vi "Client Connection Loop.vi"(11 "TCPMessaging in":refnum<class "TCPMessaging.lvclass">) -> ()   [LabVIEW 2020, in "Vecto.lvlib" / "TCPMessaging.lvclass"]
uses:
  TCPMessaging.lvclass
  Client Connection State.ctl
  TCPMessaging.lvclass/TCPMessaging.ctl
  EventLoggingService/EventLoggingService.lvclass/EventLoggingService.ctl
  Connection State.ctl
  <vilib>/Utility/error.llb/Error Cluster From Error Code.vi
  EventLogHandler/EventLogHandler.lvclass
  proto/TcpClientHello/TcpClientHello.lvlib
  Vecto.lvlib
  EventLoggingService/EventLoggingService.lvclass
  Connected Status.ctl
panel:
  out "State":T1
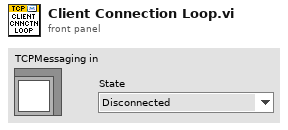
[diagram p1: front panel]
types:
  T1 = typedef "Vecto.lvlib/TCPMessaging.lvclass/Client Connection State.ctl" = enum16{"Disconnected", "Accept", "Notify Connect", "Wait Running", "Connected", "Notify Disconnect", "Reset", "Wait Stopped"}
  T2 = typedef "Vecto.lvlib/Connection State.ctl" = enum16{"Connected", "Disconnected"}
  T3 = typedef "Vecto.lvlib/Connected Status.ctl" = enum16{"Disconnected", "Connected", "Bad Config", "Not Allowed", "Server"}
  T4 = typedef "TcpClientHello.lvlib/Data.ctl" = cluster{"node_id":u32, "system":string, "cluster":string, "node_name":string, "app_version":string, "config_version":string, "config_hash":string, "node_alias":string}
  T5 = typedef "ConnectStatus.lvlib/Enumeration.ctl" = enum16{"STATUS_UNKNOWN", "STATUS_SUCCESS", "STATUS_ERROR", "STATUS_BAD_CONFIG", "STATUS_BAD_SYSTEM", "STATUS_BAD_CLUSTER", "STATUS_NOT_ALLOWED"}
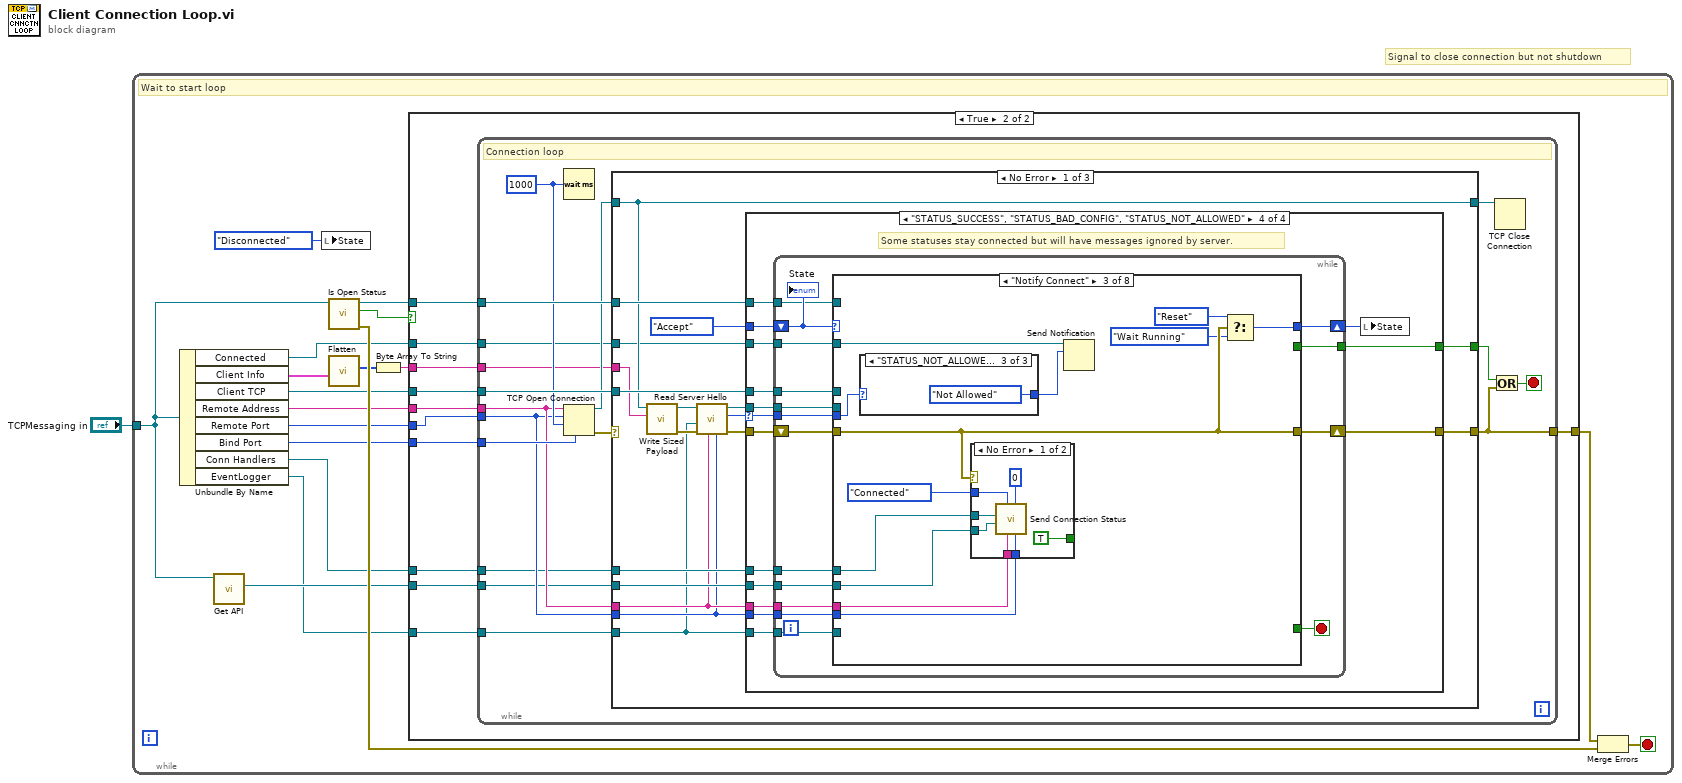
[diagram p0: block diagram]
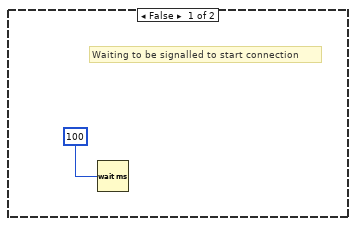
[diagram p2: hidden frame]
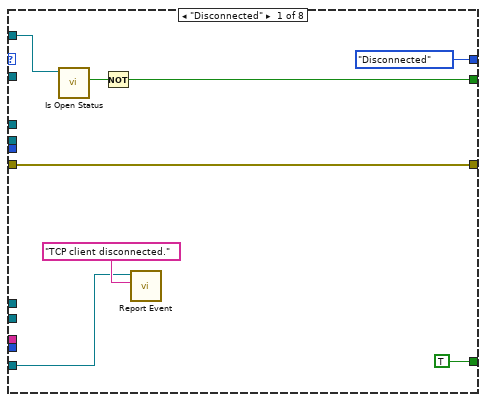
[diagram p6: hidden frame]
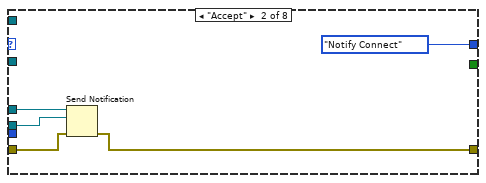
[diagram p7: hidden frame]
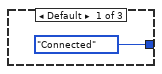
[diagram p8: hidden frame]
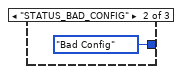
[diagram p9: hidden frame]
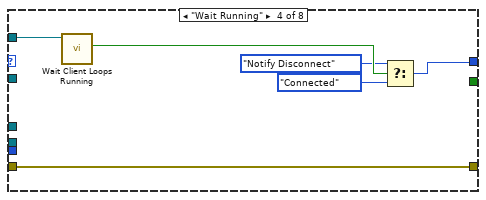
[diagram p11: hidden frame]
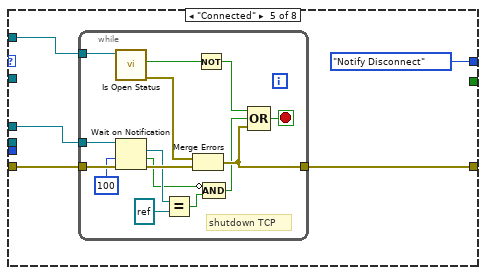
[diagram p12: hidden frame]
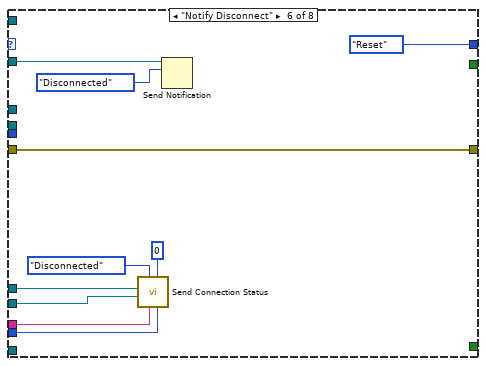
[diagram p13: hidden frame]
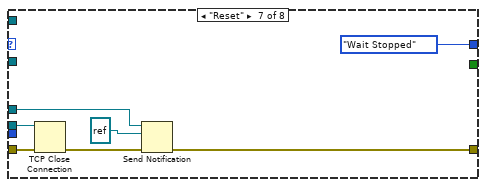
[diagram p14: hidden frame]
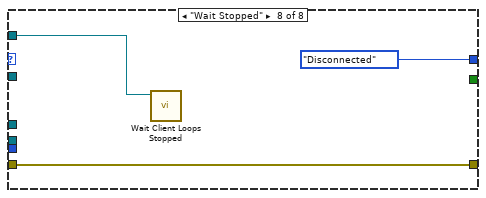
[diagram p15: hidden frame]
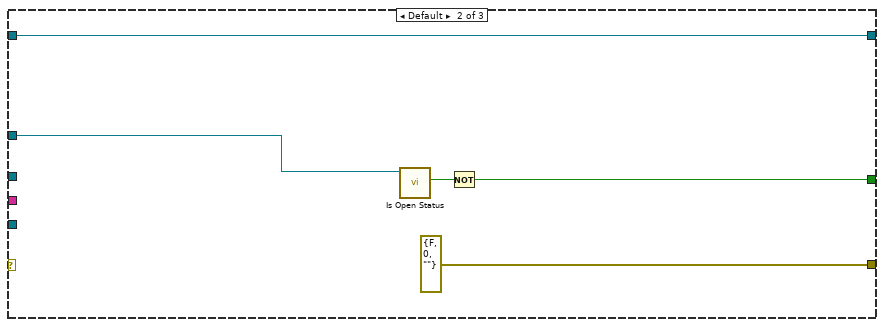
[diagram p16: hidden frame]
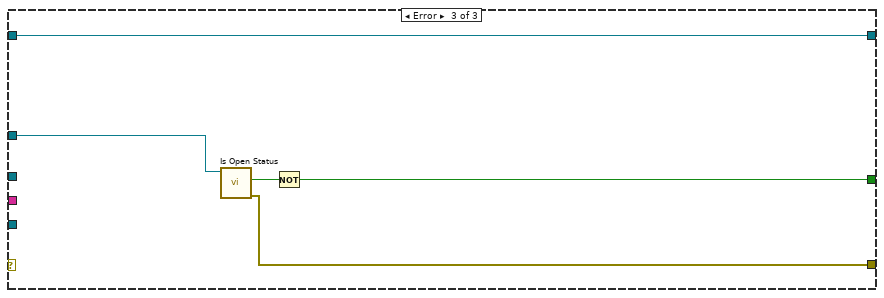
[diagram p17: hidden frame]
diagram:
  # "Signal to close connection but not shutdown"
  n1 = while {
    tunnel: "TCPMessaging in" -> [w6]
    stop <- w8 stop-if-true
    # "Wait to start loop"
    n2 = Unbundle By Name(w6) -> ("Connected"=w2:refnum<notifier>, "Client Info"=w5:T4, "Client TCP"=w13:refnum<notifier>, "Remote Address"=w18:string, "Remote Port"=w17:u16, "Bind Port"=w14:u16, "Conn Handlers"=w10:refnum<queue>, "EventLogger"=w4:refnum<class "EventLoggingService.lvclass">)
    n3 = call "Get API.vi"("TCPMessaging in"=w6) -> ("TCP Messaging API"=w9:refnum<class "TCPMessageAPI.lvclass">)  [unwired: 8 in, 2 out]
    n4 = local write "State"(Client_Connection_State."Disconnected" ("State")) -> ()
    n5 = call "Is Open Status.vi"("TCPMessaging in"=w6) -> ("error out"=w19:errorcluster, "Open"=w15:bool, "TCPMessaging out"=w16:refnum<class "TCPMessaging.lvclass">)  [unwired: 8 in]
    n6 = call "Flatten.vi"("Data"=w5) -> ("Buffer"=w12:u8[])  [unwired: 9 in, 1 out]
    n7 = Byte Array To String(unsigned byte array=w12) -> (string=w11:string)
    n8 = case shown="True" w15 {
      tunnel: w18 -> [_ w28]
      tunnel: w17 -> [_ w29]
      tunnel: w16 -> [_ w31]
      tunnel: w14 -> [_ w30]
      tunnel: w13 -> [_ w27]
      tunnel: w11 -> [_ w26]
      tunnel: w10 -> [_ w25]
      tunnel: w9 -> [_ w24]
      tunnel: [_ w23] -> w7
      tunnel: w4 -> [_ w22]
      tunnel: w2 -> [_ w21]
      frame False {
        # "Waiting to be signalled to start connection"
        n9 = Wait (ms)(milliseconds to wait=u32 100) -> ()  [unwired: 1 out]
      }
      frame True {
        n10 = while {
          tunnel: w31 -> [w44]
          tunnel: w30 -> [w47]
          tunnel: w29 -> [w37]
          tunnel: w28 -> [w38]
          tunnel: w27 -> [w45]
          tunnel: w26 -> [w39]
          tunnel: w25 -> [w36]
          tunnel: w24 -> [w35]
          tunnel: w22 -> [w34]
          tunnel: [w33] -> w23
          tunnel: w21 -> [w32]
          stop <- w48 stop-if-true
          w40 = 1000 ("timeout ms (60000)")
          # "Connection loop"
          n11 = Wait (ms)(milliseconds to wait=w40) -> ()  [unwired: 1 out]
          n12 = TCP Open Connection(address=w38, remote port or service name=w37, timeout ms (60000)=w40, local port=w47) -> (connection ID=w42:refnum<k5>, error out=w46:errorcluster)  [unwired: 1 in]
          n13 = case shown="No Error" w46 {
            tunnel: w42 -> [w62 w185 w188]
            tunnel: w45 -> [w65 _ _]
            tunnel: w44 -> [w66 w184 w191]
            tunnel: [w59 errorcluster {"status"=FALSE, "code"=0, "source"=""} ("error IO") w187] -> w33
            tunnel: [w64 w182 w189] -> w43
            tunnel: [w62 w185 w188] -> w41
            tunnel: w39 -> [w63 _ _]
            tunnel: w38 -> [w53 _ _]
            tunnel: w37 -> [w52 _ _]
            tunnel: w36 -> [w61 _ _]
            tunnel: w35 -> [w60 _ _]
            tunnel: w34 -> [w51 _ _]
            tunnel: w32 -> [w49 _ _]
            frame No Error {
              n14 = call "Write Sized Payload.vi"("Payload"=w63, "TCP in"=w62) -> ("error out"=w57:errorcluster, "TCP"=w58:refnum<k5>)  [unwired: 8 in]
              n15 = call "Read Server Hello.vi"("Port"=w52, "Address"=w53, "error in (no error)"=w57, "EventLogger"=w51, "TCP in"=w58) -> ("error out"=w56:errorcluster, "status"=w54:T5, "TCP"=w55:refnum<k5>)  [unwired: 4 in]
              n16 = case shown="\"STATUS_SUCCESS\", \"STATUS_BAD_CONFIG\", \"STATUS_NOT_ALLOWED\"" w54 {
                selector: w54 -> [_ _ _ w70]
                tunnel: w66 -> [_ _ _ w76]
                tunnel: w65 -> [_ _ _ w78]
                tunnel: [_ _ _ w73] -> w64
                tunnel: w61 -> [_ _ _ w80]
                tunnel: w60 -> [_ _ _ w81]
                tunnel: w53 -> [_ _ _ w82]
                tunnel: w52 -> [_ _ _ w83]
                tunnel: [w67 w68 w69 w74] -> w59
                tunnel: w56 -> [w67 w68 w69 w79]
                tunnel: w55 -> [_ _ _ w77]
                tunnel: w51 -> [_ _ _ w84]
                tunnel: Client_Connection_State."Accept" ("Client Connection State") -> [_ _ _ w75]
                tunnel: w49 -> [_ _ _ w71]
                frame "STATUS_BAD_SYSTEM", "STATUS_BAD_CLUSTER" {
                  # "Requires app update to resolve."
                }
                frame "STATUS_UNKNOWN" {
                }
                frame "STATUS_ERROR" {
                  # "Unknown error on server side, retry after loop delay."
                }
                frame "STATUS_SUCCESS", "STATUS_BAD_CONFIG", "STATUS_NOT_ALLOWED" {
                  # "Some statuses stay connected but will have messages ignored by server."
                  n17 = while {
                    tunnel: w84 -> [w88]
                    tunnel: w83 -> [w89]
                    tunnel: w82 -> [w90]
                    tunnel: w81 -> [w91]
                    tunnel: w80 -> [w92]
                    shift-right: [w93] -> w74
                    shift-left: w79 -> [w94]
                    tunnel: w78 -> [w96]
                    tunnel: w77 -> [w95]
                    tunnel: w76 -> [w97]
                    shift-right: [w99] -> w72
                    shift-left: w75 -> [w100]
                    tunnel: [w87] -> w73
                    tunnel: w71 -> [w86]
                    tunnel: w70 -> [w85]
                    stop <- w98 stop-if-true
                    n18 = case shown="\"Notify Connect\"" w100 {
                      tunnel: [Client_Connection_State."Disconnected" ("Client Connection State") Client_Connection_State."Notify Connect" ("Client Connection State") w118 w136 Client_Connection_State."Notify Disconnect" ("Client Connection State") Client_Connection_State."Reset" ("Client Connection State") Client_Connection_State."Wait Stopped" ("Client Connection State") Client_Connection_State."Disconnected" ("Client Connection State")] -> w99
                      tunnel: [TRUE _ _ _ _ _ _ _] -> w98
                      tunnel: w97 -> [w106 _ _ w140 w145 _ _ w180]
                      tunnel: w96 -> [_ w112 _ _ w144 _ w177 _]
                      tunnel: w95 -> [_ w110 _ _ _ _ w172 _]
                      tunnel: w94 -> [w107 w111 w125 w141 w146 w171 w176 w181]
                      tunnel: [w107 w109 w125 w141 w143 w171 w175 w181] -> w93
                      tunnel: w92 -> [_ _ w122 _ _ w169 _ _]
                      tunnel: w91 -> [_ _ w121 _ _ w168 _ _]
                      tunnel: w90 -> [_ _ w124 _ _ w167 _ _]
                      tunnel: w89 -> [_ _ w123 _ _ w166 _ _]
                      tunnel: w88 -> [w101 _ _ _ _ _ _ _]
                      tunnel: [w103 _ _ _ _ _ _ _] -> w87
                      tunnel: w86 -> [_ _ w117 _ _ w164 _ _]
                      tunnel: w85 -> [_ _ w115 _ _ _ _ _]
                      frame "Disconnected" {
                        n19 = call "Is Open Status.vi"("TCPMessaging in"=w106) -> ("Open"=w105:bool)  [unwired: 8 in, 2 out]
                        n20 = Not(x=w105) -> (.not. x?=w103:bool)
                        n21 = call "Report Event.vi"("Message"="TCP client disconnected.", "EventLoggingService in"=w101) -> ()  [unwired: 8 in, 2 out]
                      }
                      frame "Accept" {
                        n22 = Send Notification(notification=w110, notifier=w112, error in (no error)=w111) -> (error out=w109:errorcluster)  [unwired: 1 out]
                      }
                      frame "Notify Connect" {
                        n23 = case shown="\"STATUS_NOT_ALLOWED\"" w115 {
                          tunnel: [Connected_Status."Connected" ("notification") Connected_Status."Bad Config" ("notification") Connected_Status."Not Allowed" ("notification")] -> w114
                          frame Default {
                          }
                          frame "STATUS_BAD_CONFIG" {
                          }
                          frame "STATUS_NOT_ALLOWED" {
                          }
                        }
                        n24 = case shown="No Error" w125 {
                          tunnel: w122 -> [w135 _]
                          tunnel: w121 -> [w134 _]
                          tunnel: w124 -> [w133 _]
                          tunnel: w123 -> [w132 _]
                          tunnel: Connection_State."Connected" ("State") -> [w131 _]
                          tunnel: [TRUE _] -> _
                          frame No Error {
                            n25 = call "Send Connection Status.vi"("Port"=w132, "Node ID"=u32 0, "Address"=w133, "State"=w131, "TCPMessageAPI"=w134, "Conn Handlers"=w135) -> ()  [unwired: 6 in]
                          }
                          frame Error {
                          }
                        }
                        n26 = Send Notification(notification=w114, notifier=w117) -> ()  [unwired: 1 in, 2 out]
                        n27 = Select(t=Client_Connection_State."Reset", s=w125, f=Client_Connection_State."Wait Running" ("Client Connection State")) -> (s? t:f=w118:T1)
                      }
                      frame "Wait Running" {
                        n28 = call "Wait Client Loops Running.vi"("TCPMessaging in"=w140) -> ("Closing"=w138:bool)  [unwired: 8 in, 2 out]
                        n29 = Select(t=Client_Connection_State."Notify Disconnect", s=w138, f=Client_Connection_State."Connected" ("Client Connection State")) -> (s? t:f=w136:T1)
                      }
                      frame "Connected" {
                        n30 = while {
                          tunnel: w144 -> [w156]
                          tunnel: [w160] -> w143
                          tunnel: w146 -> [w161]
                          tunnel: w145 -> [w157]
                          stop <- w149 stop-if-true
                          # "shutdown TCP"
                          n31 = call "Is Open Status.vi"("TCPMessaging in"=w157) -> ("error out"=w152:errorcluster, "Open"=w158:bool)  [unwired: 8 in, 1 out]
                          n32 = Wait on Notification(notifier=w156, timeout in ms (-1)=100, error in (no error)=w161) -> (notification=w154:refnum<k5>, timed out?=w148:bool, error out=w159:errorcluster)  [unwired: 1 in, 1 out]
                          n33 = Equal?(x=w154, y=refnum<k5> refnum) -> (x = y?=w151:bool)
                          n34 = Merge Errors(w152, w159) -> (w160:errorcluster)
                          n35 = Not(x=w158) -> (.not. x?=w150:bool)
                          n36 = Compound Arithmetic op=AND(invert w148, w151) -> (w147:bool)
                          n37 = Compound Arithmetic op=OR(w150, w147, w160) -> (w149:bool)
                        }
                      }
                      frame "Notify Disconnect" {
                        n38 = call "Send Connection Status.vi"("Port"=w166, "Node ID"=u32 0, "Address"=w167, "State"=Connection_State."Disconnected", "TCPMessageAPI"=w168, "Conn Handlers"=w169) -> ()  [unwired: 6 in]
                        n39 = Send Notification(notification=Connected_Status."Disconnected", notifier=w164) -> ()  [unwired: 1 in, 2 out]
                      }
                      frame "Reset" {
                        n40 = TCP Close Connection(connection ID=w172, error in (no error)=w176) -> (error out=w173:errorcluster)  [unwired: 1 in, 1 out]
                        n41 = Send Notification(notification=refnum<k5> refnum, notifier=w177, error in (no error)=w173) -> (error out=w175:errorcluster)  [unwired: 1 out]
                      }
                      frame "Wait Stopped" {
                        n42 = call "Wait Client Loops Stopped.vi"("TCPMessaging in"=w180) -> ()  [unwired: 9 in, 2 out]
                      }
                    }
                    "State" <- w100
                  }
                  n43 = local write "State"(w72) -> ()
                }
              }
            }
            frame Default {
              n44 = call "Is Open Status.vi"("TCPMessaging in"=w184) -> ("Open"=w183:bool)  [unwired: 8 in, 2 out]
              n45 = Not(x=w183) -> (.not. x?=w182:bool)
            }
            frame Error {
              n46 = call "Is Open Status.vi"("TCPMessaging in"=w191) -> ("error out"=w187:errorcluster, "Open"=w190:bool)  [unwired: 8 in, 1 out]
              n47 = Not(x=w190) -> (.not. x?=w189:bool)
            }
          }
          n48 = Or(x=w43, y=w33) -> (x .or. y?=w48:bool)
          n49 = TCP Close Connection(connection ID=w41) -> ()  [unwired: 2 in, 2 out]
        }
      }
    }
    n50 = Merge Errors(w7, w19) -> (w8:errorcluster)
  }
